vi "Parse Datagram.vi"(4 "source address":u32, 6 "source port":u16, 7 "transfer group id":i32, 8 "error in (no error)":errorcluster, 10 "datagram":string, 11 "UDP Transceiver in":refnum<class "UDP Transceiver.lvclass">) -> (0 "error out":errorcluster, 1 "valid":bool, 2 "transfer data":string, 3 "UDP Transceiver out":refnum<class "UDP Transceiver.lvclass">, 5 "transfer id":i32)   [LabVIEW 2017, in "UDP Transceiver.lvlib" / "UDP Transceiver.lvclass"]
uses:
  UDP Transceiver.lvclass
  UDP Transceiver.lvclass/UDP Transceiver.ctl
  Throw Unknown Datagram Error.vi
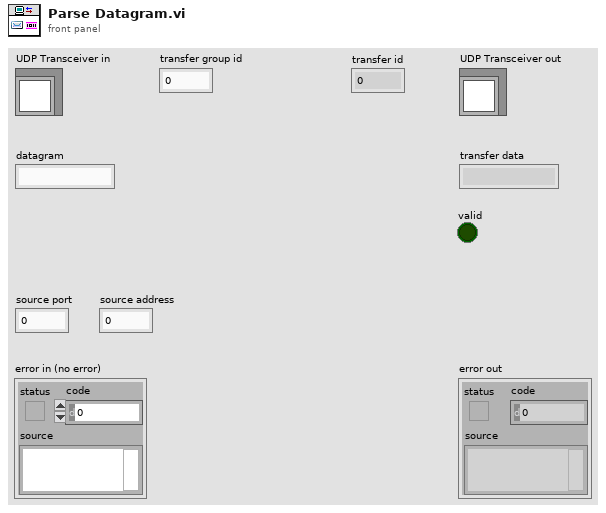
[diagram p1: front panel]
types:
  T1 = typedef "UDP Transceiver.lvlib/UDP Transceiver.lvclass/Transfer Group Parameters.ctl" = cluster{"transfers":T2[], "max size":i32, "timeout":i32}
  T2 = typedef "UDP Transceiver.lvlib/UDP Transceiver.lvclass/Transfer Parameters.ctl" = cluster{"group offset":u64, "size":u64, "address":u32, "port":u16}
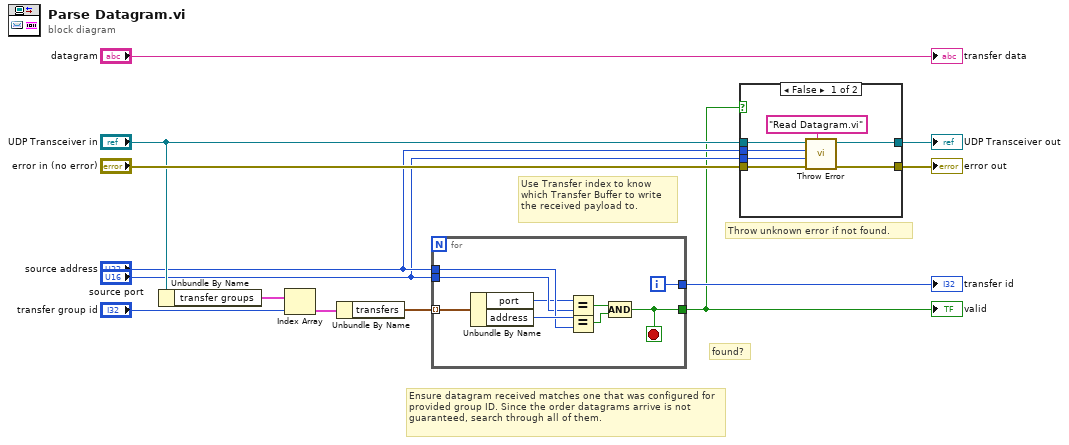
[diagram p0: block diagram]
diagram:
  # "Throw unknown error if not found."
  # "Use Transfer index to know which Transfer Buffer to write the received payload to."
  # "found?"
  # "Ensure datagram received matches one that was configured for provided group ID. Since the order datagrams arrive is not guaranteed, search through all of them."
  n1 = Unbundle By Name("UDP Transceiver in") -> ("transfer groups"=w7:T1[])
  n2 = Index Array(array=w7, index="transfer group id") -> (element=w5:T1)
  n3 = Unbundle By Name(w5) -> ("transfers"=w13:T2[])
  n4 = for {
    tunnel: w13 -> [w18] mode=indexing
    tunnel: [w20] -> w12
    tunnel: [w19] -> w2
    tunnel: "source port" -> [w15]
    tunnel: "source address" -> [w16]
    i -> [w20]
    stop <- w19 stop-if-true
    n5 = Unbundle By Name(w18) -> ("port"=w14:u16, "address"=w17:u32)
    n6 = Equal?(x=w14, y=w15) -> (x = y?=w21:bool)
    n7 = Equal?(x=w17, y=w16) -> (x = y?=w22:bool)
    n8 = Compound Arithmetic op=AND(w21, w22) -> (w19:bool)
  }
  "transfer id" <- w12
  "valid" <- w2
  n9 = case shown="False" w2 {
    tunnel: "error in (no error)" -> [w28 w30]
    tunnel: "UDP Transceiver in" -> [w29 w31]
    tunnel: [w27 w31] -> w11
    tunnel: [w26 w30] -> w10
    tunnel: "source port" -> [w24 _]
    tunnel: "source address" -> [w23 _]
    frame False {
      n10 = call-poly "Throw Error.vi"("source vi name"="Read Datagram.vi", "error in (no error)"=w28, "source port"=w24, "source address"=w23, "UDP in"=w29) -> ("error out"=w26:errorcluster, "UDP out"=w27:refnum<class "UDP Transceiver.lvclass">)  [unwired: 5 in]
    }
    frame True {
    }
  }
  "error out" <- w10
  "UDP Transceiver out" <- w11
  "transfer data" <- "datagram"
